vi "BLETesting.vi"() -> ()   [LabVIEW 2022 SP3]
uses:
  _LVsubs/MakeYourOwn/Serial_Port.xctl
  _LVsubs/MakeYourOwn/Code.xctl
  _LVsubs/MakeYourOwn/File Tree.xctl
panel:
  out "Done":bool
  in  "Settings":bool
  in  "File Tree":path(xcontrol)=path "/Users/crogers/Documents/Python Codes/SPIKE_BLE/ble_uart_Central.py"
  in  "Path":path=path "/Users/crogers/Documents/Python Codes/SPIKE_BLE/ble_uart_Central.py"
  in  "Code":string(xcontrol)="import struct\nimport time\nimport ble_CBR\nimport bluetooth\n\nclass UART_Central():\n    def __init__(self, name = '', verbose = True):\n        ble = bluetooth.BLE()\n        self.central = ble_CBR.BLESimpleCentral(ble)\n        self.not_found = False\n        self.name = name\n        \n    def printIt(self, text):\n        if verbose:\n            print(text)\n            \n    def _on_scan(self, addr_type, addr, name):\n        if addr_type is not None:\n            if self.name == '' or if self.name == name:\n                printIt(\"Found peripheral:\", addr_type, addr, name)\n                self.central.connect()\n            else:\n                printIt(\"Found unwanted peripheral:\", addr_type, addr, name)\n        else:\n            self.not_found = True\n            printIt(\"No peripheral found.\")\n\n    def _on_rx(self, v):\n        printIt(\"RX\", v)\n        \n    def connect():\n        self.central.scan(callback = on_scan)\n        self.central.on_notify(on_rx)\n\n    def wait_for_connection(self):\n        printIt('Waiting ',end = '')\n        while not self.is_connected():\n            printIt('.',end = '')\n            time.sleep(0.5)\n            if self.not_found:\n                return        \n     printIt('success')     \n    \n    def write(self, text, response = False):\n        self.central.write(payload,response)\n        \n\ncentral = UART_Central()\n\ni = 0\nwhile central.is_connected():\n    try:\n        payload = 'iteration = %d'%i\n        print(\"sending \", payload)\n        central.write(payload)\n    except:\n        print(\"TX failed\")\n    i += 1\n    time.sleep_ms(30)  # use 400 if response = True\n\nprint(\"Disconnected\")\n"
  in  "Tab Control":enum32{"Chart", "Scope", "Last lines"}(tab)=enum."Last lines"
  out "Chart":dbl(graph)
  out "Graph":dbl[](graph)
  in  "new lines":string[](array[string])=[">>> i = 0\r"]
  out "good?":bool
  in  "version":bool
  in  "Spike":bool
  in  "CtrlE":bool
  in  "Send Code":bool
  in  "clear":bool
  in  "reconnect":bool
  in  "Serial_Port":T2(xcontrol)={"session"=refnum, "PyPath"=path "/Users/crogers/GitHub/ME35_21/PythonIDE/_LVsubs/Serial/RogersSerial.py", "Processor"=enum."SPIKE", "Port"="/dev/cu.usbmodem3655376B32381", "version"="3.9"}
  in  "Console":string="\n>>> \n>>> \nWaiting ......import struct\n>>> import time\n>>> import ble_CBR\n>>> import bluetooth\n>>> class UART_Central():\n...     def __init__(self, name = '', verbose = True):\n...         ble = bluetooth.BLE()\n...         self.central = ble_CBR.BLESimpleCentral(ble)\n...         self.not_found = False\n...         self.name = name\n....     def printIt(self, text):\n...         if verbose:\n...             print(text)\n...     def _on_scan(self, addr_type, addr, name):\n...         if addr_type is not None:\n...             if self.name == '' or if self.name == name:\n...                 printIt(\"Found peripheral:\", addr_type, addr, name)\n...                 self.central.connect()\n...             else:\n...                 printIt(\"Found unwanted peripheral:\", addr_type, addr, name)\n...         else:\n...             self.not_found = True\n...             printIt(\"No peripheral found.\")\n...     def _on_rx(self, v):\n....         printIt(\"RX\", v)\n...     def connect():\n...         self.central.scan(callback = on_scan)\n...         self.central.on_notify(on_rx)\n...     def wait_for_connection(self):\n...         printIt('Waiting ',end = '')\n...         while not self.is_connected():\n...             printIt('.',end = '')\n...             time.sleep(0.5)\n...             if self.not_found:\n...                 return\n...     printIt('success')\n....     def write(self, text, response = False):\n...         self.central.write(payload,response)\n... \nTraceback (most recent call last):\n  File \"<stdin>\", line 12\nSyntaxError: invalid syntax\n>>> central = UART_Central()\nTraceback (most recent call last):\n  File \"<stdin>\", line 1, in <module>\nNameError: name 'UART_Central' isn't defined\n>>> i = 0\n>>> while central.is_connecte"
  in  "File Tree 2":path(xcontrol)=path "/Users/crogers/Documents/Python Codes/SPIKE_BLE/ble_uart_Periph.py"
  in  "Path 2":path=path "/Users/crogers/Documents/Python Codes/SPIKE_BLE/ble_uart_Periph.py"
  in  "Code 2":string(xcontrol)="import struct\nimport time\nimport ble_CBR\nimport bluetooth\n\nclass UART_Peripheral:\n    def __init__(self, name = 'MySpike'):\n        ble = bluetooth.BLE()\n        self.name = name\n        self.p = ble_CBR.BLESimplePeripheral(ble, 'UART', self.name)\n        self.p.on_write(self.on_rx)\n        \n    def on_rx(self,v):\n        print(\"RX\", v)\n        \n    def reset(self):\n        payload = struct.pack('b',Reset)\n        self.p.send(payload)   \n        \n    def wait_for_connection(self):\n        print('Waiting ',end = '')\n        while not self.is_connected():\n            print('.',end = '')\n            time.sleep(0.5)\n        self.reset()\n        print('success')     \n        \n    def is_connected(self):\n        return self.p.is_connected()\n        \n    def send(self, value):\n        if self.is_connected():\n            self.p.send(value)\n            return True\n        return False\n        \n    def fit(self, x):\n        return (0 if x < 0 else 127 if x > 127 else x)\n        \n    def sendPackage(self, text, verbose = False):\n        payload = [ord(i) for i in text]\n        if verbose:\n            print([hex(i) for i in payload])\n        return self.send(payload)\n\n    def disconnect(self):\n        self.p.disconnect()\n\nper = UART_Peripheral('Pico')\n\nper.wait_for_connection()\nper.send('test')\nper.disconnect()"
  in  "Tab Control 2":enum32{"Chart", "Scope", "Last lines"}(tab)=enum."Last lines"
  out "Chart 2":dbl(graph)
  out "Graph 2":dbl[](graph)
  in  "new lines 2":string[](array[string])=[">>> per.wait_for_connection()\r"]
  in  "Spike 2":bool
  in  "CtrlE 2":bool
  in  "version 2":bool
  in  "Send Code 2":bool
  out "good? 2":bool
  in  "reconnect 2":bool
  in  "Serial_Port 2":T2(xcontrol)={"session"=refnum, "PyPath"=path "/Users/crogers/GitHub/ME35_21/PythonIDE/_LVsubs/Serial/RogersSerial.py", "Processor"=enum."SPIKE", "Port"="/dev/cu.usbmodem101", "version"="3.9"}
  in  "Console 2":string="Traceback (most recent call last):\n  File \"<stdin>\", line 1, in <module>\n  File \"<stdin>\", line 16, in wait_for_connection\nKeyboardInterrupt: \n>>> >>> per.send('test')\nFalse\n>>> per.disconnect()\n>>> \n>>> \n>>> import struct\n>>> import time\n>>> import ble_CBR\n>>> import bluetooth\n>>> class UART_Peripheral:\n...     def __init__(self, name = 'MySpike'):\n...         ble = bluetooth.BLE()\n...         self.name = name\n...         self.p = ble_CBR.BLESimplePeripheral(ble, 'UART', self.name)\n...         self.p.on_write(self.on_rx)\n...     def on_rx(self,v):\n...         print(\"RX\", v)\n...     def reset(self):\n...         payload = struct.pack('b',Reset)\n...         self.p.send(payload)\n...     def wait_for_connection(self):\n...         print('Waiting ',end = '')\n...         while not self.is_connected():\n...             print('.',end = '')\n...             time.sleep(0.5)\n...         self.reset()\n...         print('success')\n...     def is_connected(self):\n...         return self.p.is_connected()\n...     def send(self, value):\n...         if self.is_connected():\n...             self.p.send(value)\n...             return True\n...         return False\n...     def fit(self, x):\n...         return (0 if x < 0 else 127 if x > 127 else x)\n...     def sendPackage(self, text, verbose = False):\n...         payload = [ord(i) for i in text]\n...         if verbose:\n...             print([hex(i) for i in payload])\n...         return self.send(payload)\n...     def disconnect(self):\n...         self.p.disconnect()\n... \n>>> per = UART_Peripheral('Pico')\nsetup as uart\nStarting advertising\n>>> per.wait_for_connection()\n>>> while central.is_connecte............................."
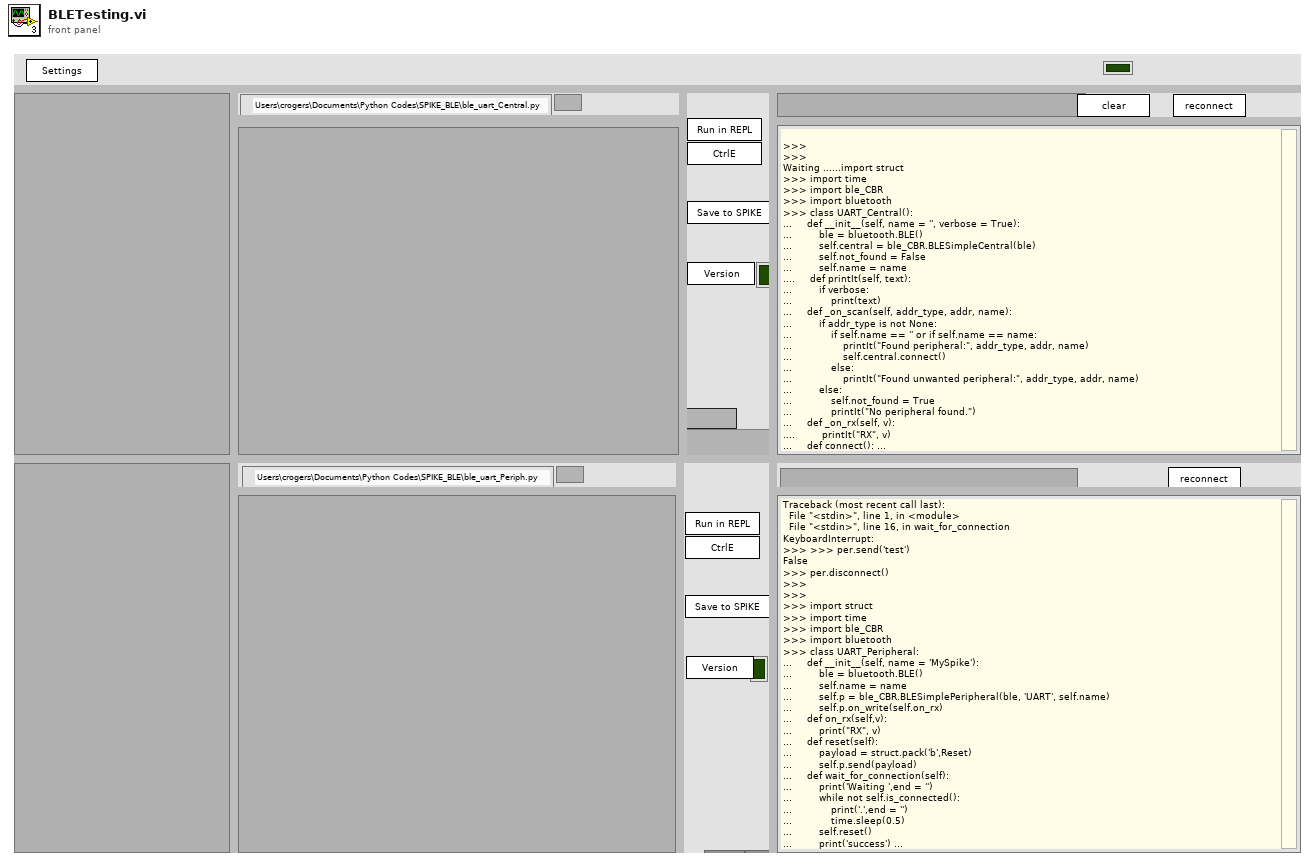
[diagram p1: front panel]
types:
  T1 = typedef "Processors.ctl" = enum16{"SPIKE", "Pi", "Pi_ssh", "OpenMV", "Dunio"}
  T2 = cluster{"session":refnum<k35>, "PyPath":path, "Processor":T1, "Port":string, "version":string}
  T3 = typedef "Preferences.ctl" = cluster{"python":string, "arduino CLI":path, "pythonCodes":cluster{"pythonCode":path, "Color":u32}[], "FontSize":u8, "Text Colors":cluster{"Quote":u32, "function":u32, "Python":u32, "Comment":u32, "Triple Quote":u32, "Text":u32}, "SSH Logins":cluster{"IP Address":string, "Username":string, "password":string}[], "packet size":u8}
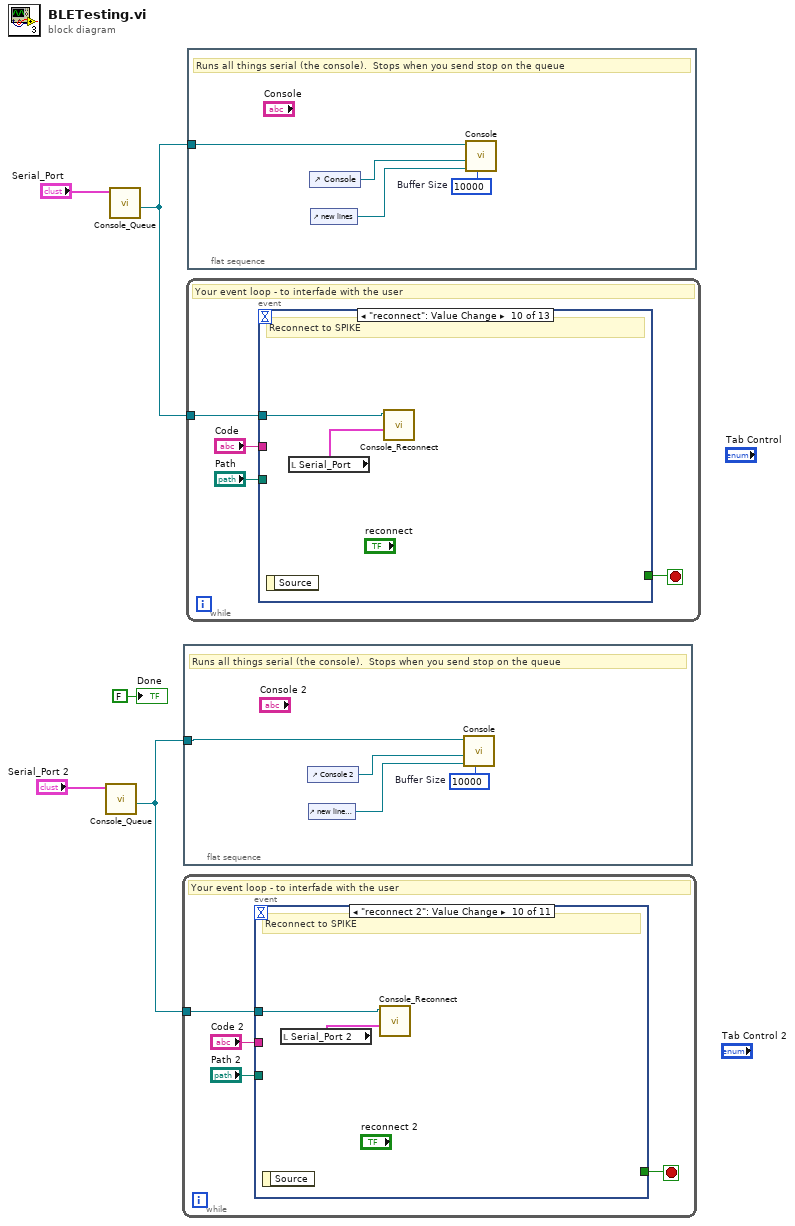
[diagram p0: block diagram]
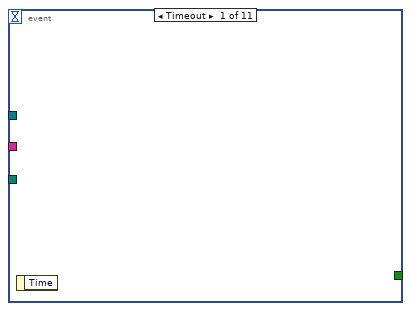
[diagram p2: hidden frame]
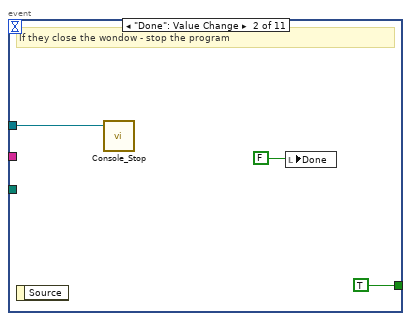
[diagram p3: hidden frame]
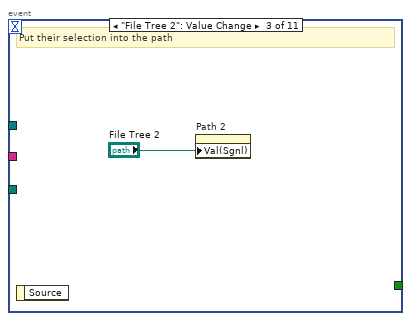
[diagram p4: hidden frame]
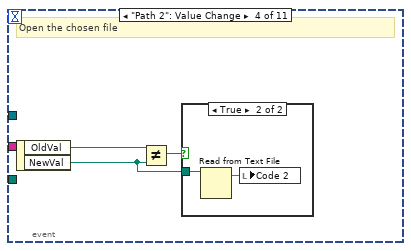
[diagram p5: hidden frame]
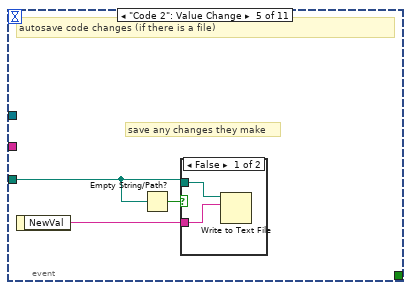
[diagram p7: hidden frame]
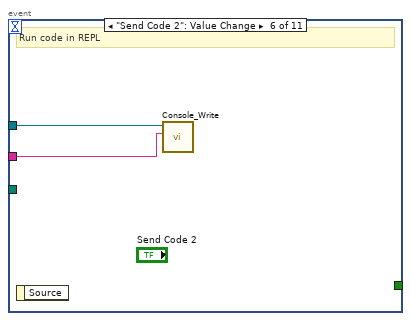
[diagram p9: hidden frame]
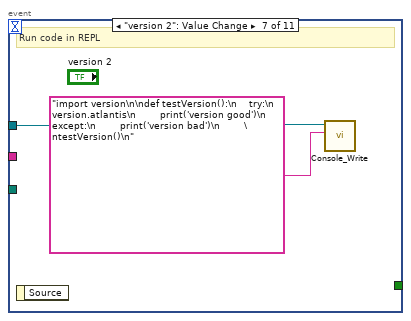
[diagram p10: hidden frame]
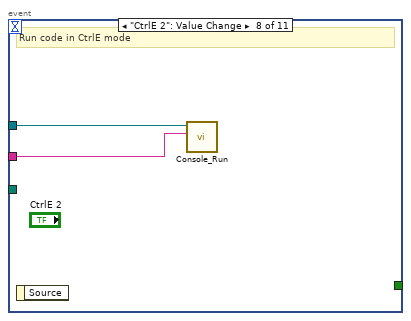
[diagram p11: hidden frame]
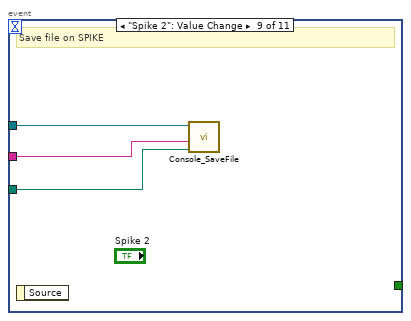
[diagram p12: hidden frame]
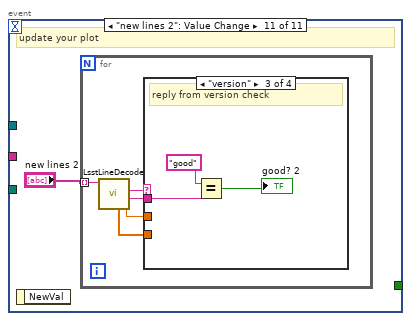
[diagram p13: hidden frame]
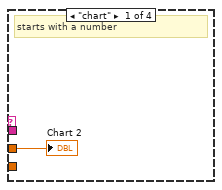
[diagram p14: hidden frame]
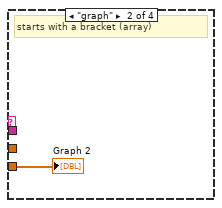
[diagram p15: hidden frame]
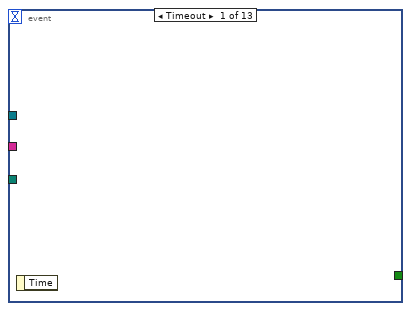
[diagram p17: hidden frame]
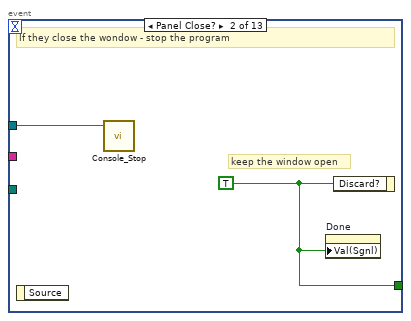
[diagram p18: hidden frame]
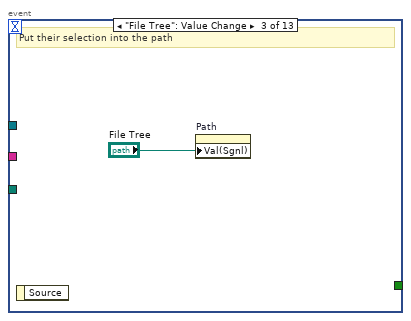
[diagram p19: hidden frame]
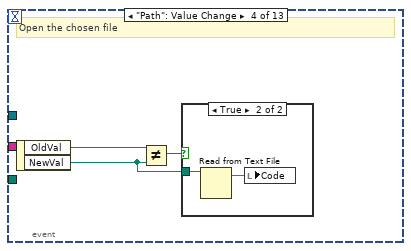
[diagram p20: hidden frame]
diagram:
  n1 = call "Console_Queue.vi"("Serial_Port"="Serial_Port 2") -> ("Queue out"=w2:refnum<queue>)  [unwired: 9 in, 1 out]
  n2 = call "Console_Queue.vi"("Serial_Port"="Serial_Port") -> ("Queue out"=w5:refnum<queue>)  [unwired: 9 in, 1 out]
  n3 = while {
    tunnel: w2 -> [w8]
    stop <- w9 stop-if-true
    # "Your event loop - to interfade with the user"
    n4 = event shown="[9] \"reconnect 2\": Value Change" {
      selector: _ -> [_ _ _ _ _ _ _ _ _ _ _]
      dyn-events: _ -> [_ _ _ _ _ _ _ _ _ _ _]
      timeout: _ -> [_ _ _ _ _ _ _ _ _ _ _]
      tunnel: [_ TRUE ("Discard?") _ _ _ _ _ _ _ _ _] -> w9
      tunnel: w8 -> [_ w11 _ _ _ w25 w27 w29 w32 w34 _]
      tunnel: "Path 2" -> [_ _ _ _ w19 _ _ _ w30 _ _]
      tunnel: "Code 2" -> [_ _ _ _ _ w24 _ w28 w31 _ _]
      event Timeout {
        n5 = event-data() -> ()  [unwired: 1 in, 1 out]
      }
      event "Done": Value Change {
        # "If they close the wondow - stop the program"
        n6 = event-data() -> ()  [unwired: 1 in, 1 out]
        n7 = call "Console_Stop.vi"("Queue in"=w11) -> ()  [unwired: 11 in]
        n8 = local write "Done"(FALSE ("Done")) -> ()
      }
      event "File Tree 2": Value Change {
        # "Put their selection into the path"
        n9 = event-data() -> ()  [unwired: 1 in, 1 out]
        n10 = property on="Path 2" class="Path"("Val(Sgnl)"="File Tree 2") -> ()  [unwired: 2 in, 2 out]
      }
      event "Path 2": Value Change {
        # "Open the chosen file"
        n11 = event-data() -> ("OldVal"=w16:path, "NewVal"=w14:path)  [unwired: 1 in]
        n12 = Not Equal?(x=w16, y=w14) -> (x != y?=w15:bool)
        n13 = case shown="True" w15 {
          tunnel: w14 -> [_ w18]
          frame False {
          }
          frame True {
            n14 = Read from Text File(file (use dialog)=w18) -> (text=w17:string)  [unwired: 3 in, 3 out]
            n15 = local write "Code 2"(w17) -> ()
          }
        }
      }
      event "Code 2": Value Change {
        # "save any changes they make"
        # "autosave code changes (if there is a file)"
        n16 = event-data() -> ("NewVal"=w21:string)  [unwired: 1 in]
        n17 = Empty String/Path?(string/path=w19) -> (empty?=w20:bool)
        n18 = case shown="False" w20 {
          tunnel: w21 -> [w23 _]
          tunnel: w19 -> [w22 _]
          frame False {
            n19 = Write to Text File(file (use dialog)=w22, text=w23) -> ()  [unwired: 2 in, 3 out]
          }
          frame True {
          }
        }
      }
      event "Send Code 2": Value Change {
        # "Run code in REPL"
        n20 = event-data() -> ()  [unwired: 1 in, 1 out]
        n21 = call "Console_Write.vi"("Code"=w24, "Queue in"=w25) -> ()  [unwired: 10 in]
      }
      event "version 2": Value Change {
        # "Run code in REPL"
        n22 = event-data() -> ()  [unwired: 1 in, 1 out]
        n23 = call "Console_Write.vi"("Code"="import version\n\ndef testVersion():\n    try:\n        version.atlantis\n        print('version good')\n    except:\n        print('version bad')\n        \ntestVersion()\n", "Queue in"=w27) -> ()  [unwired: 10 in]
      }
      event "CtrlE 2": Value Change {
        # "Run code in CtrlE mode"
        n24 = event-data() -> ()  [unwired: 1 in, 1 out]
        n25 = call "Console_Run.vi"("Code"=w28, "Queue in"=w29) -> ()  [unwired: 10 in]
      }
      event "Spike 2": Value Change {
        # "Save file on SPIKE"
        n26 = event-data() -> ()  [unwired: 1 in, 1 out]
        n27 = call "Console_SaveFile.vi"("Path"=w30, "Code"=w31, "Queue in"=w32) -> ()  [unwired: 9 in]
      }
      event "reconnect 2": Value Change {
        # "Reconnect to SPIKE"
        n28 = event-data() -> ()  [unwired: 1 in, 1 out]
        n29 = local read "Serial_Port 2"() -> (w33:T2)
        n30 = call "Console_Reconnect.vi"("Python"=w33, "Queue in"=w34) -> ()  [unwired: 10 in]
      }
      event "new lines 2": Value Change {
        # "update your plot"
        n31 = event-data() -> ()  [unwired: 1 in, 1 out]
        n32 = for {
          tunnel: "new lines 2" -> [w36] mode=indexing
          n33 = call "LsstLineDecode.vi"("new lines"=w36) -> ("Chart"=w39:dbl, "payload"=w37:string, "cmd"=w40:string, "Graph"=w38:dbl[])  [unwired: 6 in, 1 out]
          n34 = case shown="\"version\"" w40 {
            tunnel: w39 -> [w41 _ _ _]
            tunnel: w38 -> [_ w42 _ _]
            tunnel: w37 -> [_ _ w45 _]
            frame "chart" {
              # "starts with a number"
              "Chart 2" <- w41
            }
            frame "graph" {
              # "starts with a bracket (array)"
              "Graph 2" <- w42
            }
            frame "version" {
              # "reply from version check"
              n35 = Equal?(x="good", y=w45) -> (x = y?=→"good? 2":bool)
            }
            frame Default {
              # "Some command"
            }
          }
        }
      }
    }
  }
  n36 = flat-sequence {
    tunnel: w2 -> [w46]
    frame #0 {
      w48 = 10000  # Buffer Size
      # "Runs all things serial (the console).  Stops when you send stop on the queue"
      n37 = control-ref of="Console 2"() -> (w49:refnum<vi>)
      n38 = control-ref of="new lines 2"() -> (w47:refnum<vi>)
      n39 = call "Console.vi"("Buffer Size"=w48, "Last Lines"=w47, "Remote Console"=w49, "Queue in"=w46) -> ()  [unwired: 8 in]
    }
  }
  n40 = while {
    tunnel: w5 -> [w52]
    stop <- w53 stop-if-true
    # "Your event loop - to interfade with the user"
    n41 = event shown="[9] \"reconnect\": Value Change" {
      selector: _ -> [_ _ _ _ _ _ _ _ _ _ _ _ _]
      dyn-events: _ -> [_ _ _ _ _ _ _ _ _ _ _ _ _]
      timeout: _ -> [_ _ _ _ _ _ _ _ _ _ _ _ _]
      tunnel: [_ w54 _ _ _ _ _ _ _ _ _ _ _] -> w53
      tunnel: w52 -> [_ w55 _ _ _ w68 w70 w72 w75 w77 w78 _ _]
      tunnel: "Path" -> [_ _ _ _ w62 _ _ _ w73 _ _ _ _]
      tunnel: "Code" -> [_ _ _ _ _ w67 _ w71 w74 _ _ _ _]
      event Timeout {
        n42 = event-data() -> ()  [unwired: 1 in, 1 out]
      }
      event Panel Close? {
        w54 = TRUE ("Discard?")
        # "keep the window open"
        # "If they close the wondow - stop the program"
        n43 = event-data() -> ()  [unwired: 1 in, 1 out]
        n44 = call "Console_Stop.vi"("Queue in"=w55) -> ()  [unwired: 11 in]
        n45 = property on="Done" class="Bool (strict)"("Val(Sgnl)"=w54) -> ()  [unwired: 2 in, 2 out]
        n46 = event-data("Discard?"=w54) -> ()  [unwired: 1 in, 1 out]
      }
      event "File Tree": Value Change {
        # "Put their selection into the path"
        n47 = event-data() -> ()  [unwired: 1 in, 1 out]
        n48 = property on="Path" class="Path"("Val(Sgnl)"="File Tree") -> ()  [unwired: 2 in, 2 out]
      }
      event "Path": Value Change {
        # "Open the chosen file"
        n49 = event-data() -> ("OldVal"=w59:path, "NewVal"=w57:path)  [unwired: 1 in]
        n50 = Not Equal?(x=w59, y=w57) -> (x != y?=w58:bool)
        n51 = case shown="True" w58 {
          tunnel: w57 -> [_ w61]
          frame False {
          }
          frame True {
            n52 = Read from Text File(file (use dialog)=w61) -> (text=w60:string)  [unwired: 3 in, 3 out]
            n53 = local write "Code"(w60) -> ()
          }
        }
      }
      event "Code": Value Change {
        # "save any changes they make"
        # "autosave code changes (if there is a file)"
        n54 = event-data() -> ("NewVal"=w64:string)  [unwired: 1 in]
        n55 = Empty String/Path?(string/path=w62) -> (empty?=w63:bool)
        n56 = case shown="False" w63 {
          tunnel: w64 -> [w66 _]
          tunnel: w62 -> [w65 _]
          frame False {
            n57 = Write to Text File(file (use dialog)=w65, text=w66) -> ()  [unwired: 2 in, 3 out]
          }
          frame True {
          }
        }
      }
      event "Send Code": Value Change {
        # "Run code in REPL"
        n58 = event-data() -> ()  [unwired: 1 in, 1 out]
        n59 = call "Console_Write.vi"("Code"=w67, "Queue in"=w68) -> ()  [unwired: 10 in]
      }
      event "version": Value Change {
        # "Run code in REPL"
        n60 = event-data() -> ()  [unwired: 1 in, 1 out]
        n61 = call "Console_Write.vi"("Code"="import version\n\ndef testVersion():\n    try:\n        version.atlantis\n        print('version good')\n    except:\n        print('version bad')\n        \ntestVersion()\n", "Queue in"=w70) -> ()  [unwired: 10 in]
      }
      event "CtrlE": Value Change {
        # "Run code in CtrlE mode"
        n62 = event-data() -> ()  [unwired: 1 in, 1 out]
        n63 = call "Console_Run.vi"("Code"=w71, "Queue in"=w72) -> ()  [unwired: 10 in]
      }
      event "Spike": Value Change {
        # "Save file on SPIKE"
        n64 = event-data() -> ()  [unwired: 1 in, 1 out]
        n65 = call "Console_SaveFile.vi"("Path"=w73, "Code"=w74, "Queue in"=w75) -> ()  [unwired: 9 in]
      }
      event "reconnect": Value Change {
        # "Reconnect to SPIKE"
        n66 = event-data() -> ()  [unwired: 1 in, 1 out]
        n67 = local read "Serial_Port"() -> (w76:T2)
        n68 = call "Console_Reconnect.vi"("Python"=w76, "Queue in"=w77) -> ()  [unwired: 10 in]
      }
      event "clear": Value Change {
        # "Reconnect to SPIKE"
        n69 = event-data() -> ()  [unwired: 1 in, 1 out]
        n70 = Enqueue Element At Opposite End(queue=w78, element="clear") -> ()  [unwired: 2 in, 3 out]
      }
      event "Settings": Value Change {
        # "Edit settings"
        n71 = event-data() -> ()  [unwired: 1 in, 1 out]
        n72 = call "Preferences.vi"() -> ("Preferences out"=w80:T3)  [unwired: 10 in, 1 out]
        n73 = call "Settings.vi"("Prefs"=w80) -> ()  [unwired: 10 in, 1 out]
      }
      event "new lines": Value Change {
        # "update your plot"
        n74 = event-data() -> ()  [unwired: 1 in, 1 out]
        n75 = for {
          tunnel: "new lines" -> [w82] mode=indexing
          n76 = call "LsstLineDecode.vi"("new lines"=w82) -> ("Chart"=w85:dbl, "payload"=w83:string, "cmd"=w86:string, "Graph"=w84:dbl[])  [unwired: 6 in, 1 out]
          n77 = case shown="\"version\"" w86 {
            tunnel: w85 -> [w87 _ _ _]
            tunnel: w84 -> [_ w88 _ _]
            tunnel: w83 -> [_ _ w91 _]
            frame "chart" {
              # "starts with a number"
              "Chart" <- w87
            }
            frame "graph" {
              # "starts with a bracket (array)"
              "Graph" <- w88
            }
            frame "version" {
              # "reply from version check"
              n78 = Equal?(x="good", y=w91) -> (x = y?=→"good?":bool)
            }
            frame Default {
              # "Some command"
            }
          }
        }
      }
    }
  }
  n79 = flat-sequence {
    tunnel: w5 -> [w92]
    frame #0 {
      w94 = 10000  # Buffer Size
      # "Runs all things serial (the console).  Stops when you send stop on the queue"
      n80 = control-ref of="Console"() -> (w95:refnum<vi>)
      n81 = control-ref of="new lines"() -> (w93:refnum<vi>)
      n82 = call "Console.vi"("Buffer Size"=w94, "Last Lines"=w93, "Remote Console"=w95, "Queue in"=w92) -> ()  [unwired: 8 in]
    }
  }
  "Done" <- FALSE ("Done")
